vi "Initialise.vi"(8 "error in (no error)":errorcluster, 9 "gaussian stdev (elements)":dbl=7.0, 10 "start value":dbl, 11 "number of elements (max 2048)":i32=50) -> (0 "error out":errorcluster, 3 "parameter cluster":T1)   [LabVIEW 2015, in "RealTimeFilter.lvlib"]
uses:
  RealTimeFilter.lvlib
  TypeDefs/Parameters.ctl
  <vilib>/Analysis/baseanly.llb/Mean (DBL).vi
  <vilib>/Analysis/NI_AALBase.lvlib
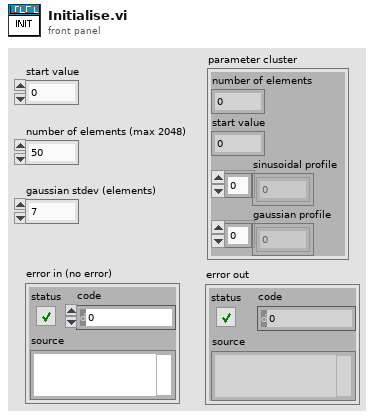
[diagram p1: front panel]
types:
  T1 = typedef "RealTimeFilter.lvlib/Parameters.ctl" = cluster{"number of elements":i32, "start value":dbl, "sinusoidal profile":dbl[], "gaussian profile":dbl[]}
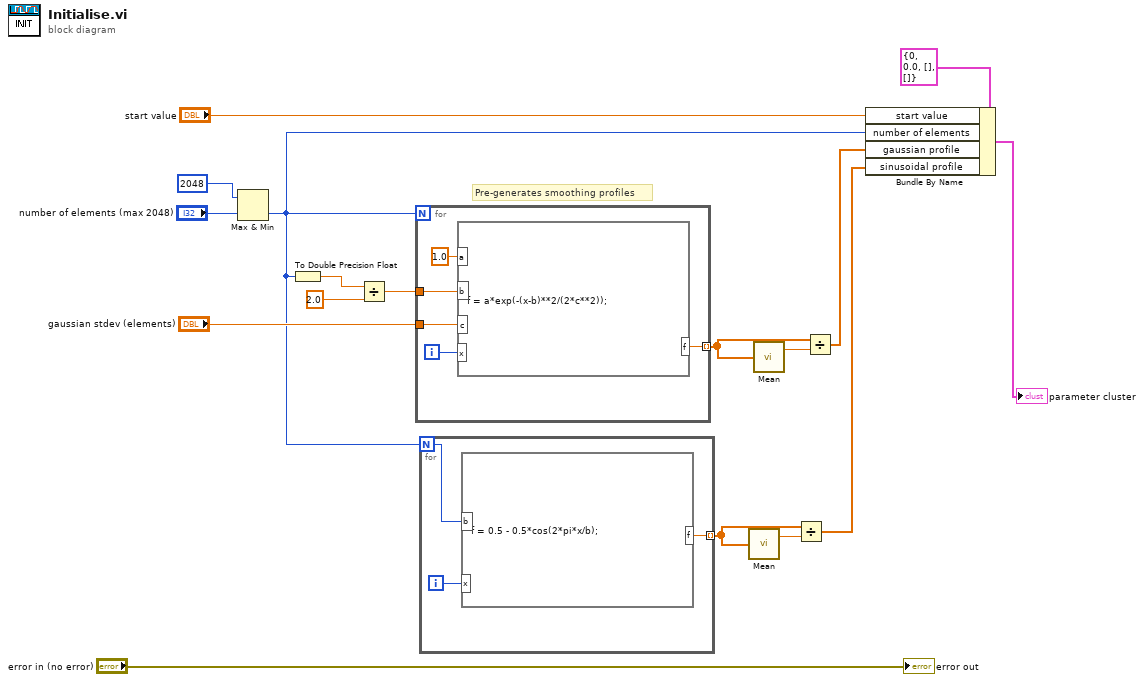
[diagram p0: block diagram]
diagram:
  # "Pre-generates smoothing profiles"
  n1 = Max & Min(x=2048, y="number of elements (max 2048)") -> (min(x,y)=w2:i32)  [unwired: 1 out]
  n2 = To Double Precision Float(number=w2) -> (double precision float=w16:dbl)
  n3 = Divide(x=w16, y=2.0 ("input variable")) -> (x/y=w12:dbl)
  n4 = for {
    N: w2 -> [_]
    tunnel: [w20] -> w13 mode=indexing
    tunnel: "gaussian stdev (elements)" -> [w19]
    tunnel: w12 -> [w18]
    i -> [w21]
    n5 = formula code="f = a*exp(-(x-b)**2/(2*c**2));"("a"=1.0 ("input variable"), "b"=w18, "c"=w19, "x"=w21) -> ("f"=w20:dbl)
  }
  n6 = for {
    N: w2 -> [w23]
    tunnel: [w24] -> w10 mode=indexing
    i -> [w25]
    n7 = formula code="f = 0.5 - 0.5*cos(2*pi*x/b);"("b"=w23, "x"=w25) -> ("f"=w24:dbl)
  }
  n8 = call-poly <vilib>:"Mean.vi"("X"=w10) -> ("mean"=w11:dbl)  [unwired: 1 out]
  n9 = call-poly <vilib>:"Mean.vi"("X"=w13) -> ("mean"=w14:dbl)  [unwired: 1 out]
  n10 = Divide(x=w10, y=w11) -> (x/y=w6:dbl[])
  n11 = Divide(x=w13, y=w14) -> (x/y=w7:dbl[])
  n12 = Bundle By Name(cluster=T1 {"number of elements"=0, "start value"=0.0, "sinusoidal profile"=[], "gaussian profile"=[]} ("parameter cluster"), "start value"="start value", "number of elements"=w2, "gaussian profile"=w7, "sinusoidal profile"=w6) -> (→"parameter cluster":T1)
  "error out" <- "error in (no error)"
